vi "MakeItemVisible.vi"(0 "MC ListBox Ref In":refnum<vi>, 5 "Item Index":i32, 11 "Error In":errorcluster) -> (4 "MC ListBox Ref Out":refnum<vi>, 15 "Error Out":errorcluster)   [LabVIEW 2016, in "Drona.lvlib" / "ControlValue.lvlib" / "StimulusMCListbox.lvlib"]
doc: "Make the specified item index to visible in the Multi column listbox control."
uses:
  StimulusMCListbox.lvlib
  <vilib>/Utility/miscctls.llb/LVRowAndColumnUnsignedTypeDef.ctl
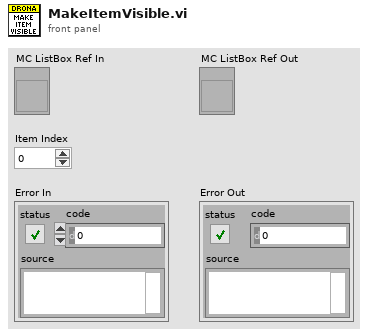
[diagram p1: front panel]
types:
  T1 = typedef "LVRowAndColumnUnsignedTypeDef.ctl" = cluster{"Row":u32, "Column":u32}
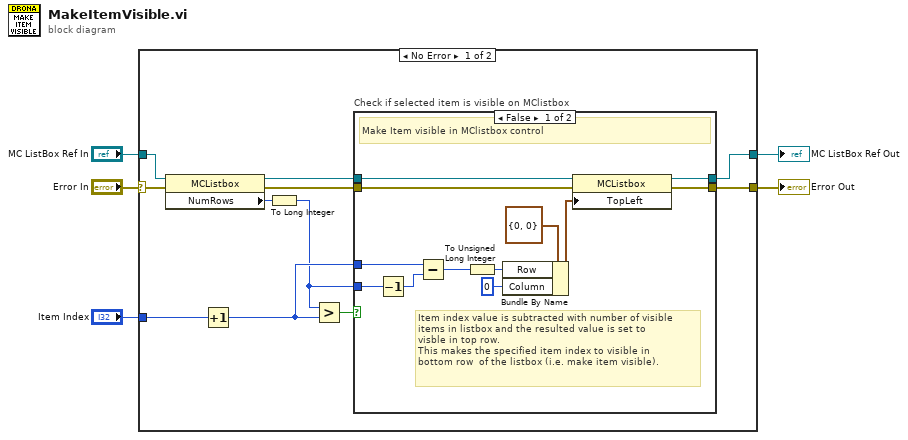
[diagram p0: block diagram]
diagram:
  n1 = case shown="No Error" "Error In" {
    selector: "Error In" -> [w6 w31]
    tunnel: [w16 w32] -> w5
    tunnel: "Item Index" -> [w15 _]
    tunnel: [w10 w31] -> w3
    tunnel: "MC ListBox Ref In" -> [w8 w32]
    frame No Error {
      n2 = property class="MCListbox"(reference=w8, error in=w6) -> (reference out=w11:refnum<vi>, error out=w7:errorcluster, "NumRows"=w9:u32)
      n3 = Increment(x=w15) -> (x+1=w14:i32)
      n4 = To Long Integer(number=w9) -> (32bit integer=w12:i32)
      n5 = Greater?(x=w12, y=w14) -> (0:w13:bool)
      n6 = case "Check if selected item is visible on MClistbox" shown="False" w13 {
        tunnel: w7 -> [w28 w30]
        tunnel: [w27 w30] -> w10
        tunnel: w11 -> [w26 w29]
        tunnel: w14 -> [w25 _]
        tunnel: w12 -> [w24 _]
        tunnel: [w22 w29] -> w16
        frame False {
          # "Item index value is subtracted with number of visible \nitems in listbox and the resulted value is set to \nvisble in top row. \nThis makes the specified item index to visible in \nbottom row  of the listbox (i.e. make item visible)."
          # "Make Item visible in MClistbox control"
          n7 = Decrement(x=w24) -> (x-1=w23:i32)
          n8 = Subtract(x=w25, y=w23) -> (x-y=w20:i32)
          n9 = To Unsigned Long Integer(number=w20) -> (unsigned 32bit integer=w19:u32)
          n10 = Bundle By Name(cluster=T1 {"Row"=0, "Column"=0} ("Top Left Visible Cell"), "Row"=w19, "Column"=u32 0) -> (w17:T1)
          n11 = property class="MCListbox"(reference=w26, error in=w28, "TopLeft"=w17) -> (reference out=w22:refnum<vi>, error out=w27:errorcluster)
        }
        frame True {
          # "Specidied item index is already visible\non MClistbox"
        }
      }
    }
    frame Error {
    }
  }
  "MC ListBox Ref Out" <- w5
  "Error Out" <- w3
